vi "QMH_handError_queue.vi"(6 "Queue_Ref":T1, 8 "error in (no error)":errorcluster) -> (0 "error out":errorcluster)   [LabVIEW 2021, in "Framework_lib.lvlib"]
uses:
  Framework_lib.lvlib
  QMH_references_enum.ctl
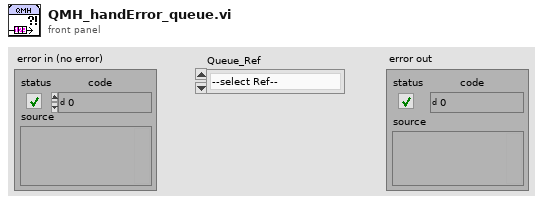
[diagram p1: front panel]
types:
  T1 = typedef "Framework_lib.lvlib/QMH_references_enum.ctl" = enum16{"--select Ref--", "Consumer_SUT", "Consumer_Annot", "Compute_Results"}
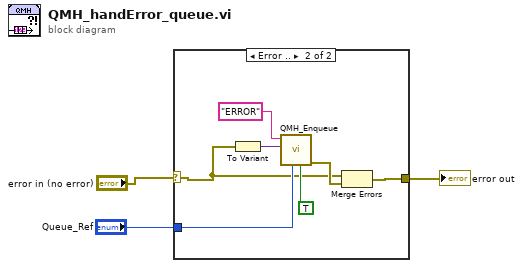
[diagram p0: block diagram]
diagram:
  n1 = case shown="Error .." "error in (no error)" {
    selector: "error in (no error)" -> [w4 w5]
    tunnel: [w4 w6] -> w2
    tunnel: "Queue_Ref" -> [_ w10]
    frame No Error {
    }
    frame Error {
      n2 = To Variant(anything=w5) -> (Variant=w9:variant)
      n3 = call "QMH_Enqueue.vi"("Priority? (F)"=TRUE, "Queue_Ref"=w10, "Payload"=w9, "Message"="ERROR") -> ("error out"=w11:errorcluster)  [unwired: 7 in]
      n4 = Merge Errors(w5, w11) -> (w6:errorcluster)
    }
  }
  "error out" <- w2
